vi "temperature-smoke-servo-control.vi"() -> ()   [LabVIEW 2019]
doc: "This example demonstrates how to read N channels of analog input from a LINX device."
uses:
  <vilib>/MakerHub/LINX/Public/Peripherals/Analog/Analog Read N Chans.vi
  <vilib>/MakerHub/LINX/Public/Peripherals/Analog/Analog Read 1 Chan.vi
  <vilib>/MakerHub/LINX/Public/Peripherals/Digital/Digital Write 1 Chan.vi
  <vilib>/MakerHub/LINX/Private/Local IO/LinxAnalogRead.vi
  <vilib>/MakerHub/LINX/Public/Utilities/Check Channel.vi
  <vilib>/MakerHub/LINX/Public/Peripherals/Digital/Digital Write N Chans.vi
  <vilib>/MakerHub/LINX/Private/Local IO/LinxDigitalWrite.vi
  <vilib>/MakerHub/LINX/Public/Utilities/Open Serial.vi
  <vilib>/MakerHub/LINX/Public/Sensors/Motion/Servo/Servo Open One Channel.vi
  <vilib>/MakerHub/LINX/Private/Utilties/Generate Error.vi
  <vilib>/imath/engines/lvmath2/RunTimeEngine/Managers/WorkSpace/UID Generator.vi
  <vilib>/imath/engines/lvmath2/RunTimeEngine/RunTimeType/NIMS_RunTimeType_From StrictType (excl LVString).vi
  <instcachedir>/0/NIMS_RunTimeType_From StrictType (excl LVString)_6DA94F09978249AAA8963F8D3C6FF051.lvgen/NIMS_RunTimeType_From StrictType (excl LVString)_6DA94F09978249AAA8963F8D3C6FF051_000.vi
  <vilib>/imath/engines/lvmath2/RunTimeEngine/LocalVariableDefStatement/MC_LocalVariableDefStatement_Display.vi
  <vilib>/imath/engines/lvmath2/RunTimeEngine/ArithmeticOperatorToken/NIMS_ArithmeticOperator_power(S).vi
  <instcachedir>/0/NIMS_ArithmeticOperator_power(S)_79C546042FF149A69349E20DC63C3C5B.lvgen/NIMS_ArithmeticOperator_power(S)_79C546042FF149A69349E20DC63C3C5B_014.vi
  <vilib>/imathl/engines/lvmath/Functions/Error Handling/Create Error.vi
  <vilib>/imath/engines/lvmath2/RunTimeEngine/Managers/SymbolTable/Clear UID.vi
  <vilib>/imath/engines/lvmath2/RunTimeEngine/NodeEndStatement/NIMS_NodeEndStatement_Output.vi
  <instcachedir>/0/NIMS_NodeEndStatement_Output_53EC0D466D134D7ABD903AC30B43404B.lvgen/NIMS_NodeEndStatement_Output_53EC0D466D134D7ABD903AC30B43404B_001.vi
  <instcachedir>/0/NIMS_NodeEndStatement_Output_53EC0D466D134D7ABD903AC30B43404B.lvgen/NIMS_NodeEndStatement_Output_53EC0D466D134D7ABD903AC30B43404B_008.vi
  <vilib>/imath/engines/lvmath2/RunTimeEngine/ErrorHandling/NIMS_Finalize Error.vi
  <instcachedir>/0/NIMS_NodeEndStatement_Output_53EC0D466D134D7ABD903AC30B43404B.lvgen/NIMS_NodeEndStatement_Output_53EC0D466D134D7ABD903AC30B43404B_010.vi
  <instcachedir>/0/NIMS_NodeEndStatement_Output_53EC0D466D134D7ABD903AC30B43404B.lvgen/NIMS_NodeEndStatement_Output_53EC0D466D134D7ABD903AC30B43404B_009.vi
  <vilib>/MakerHub/LINX/Public/Sensors/Motion/Servo/Servo Set Pulse Width One Channel.vi
  <vilib>/MakerHub/LINX/Public/Sensors/Motion/Servo/Servo Close One Channel.vi
  <vilib>/MakerHub/LINX/LMH-LINX.lvlib
  <vilib>/ptbypt/NI_PtbyPt.lvlib
  <vilib>/imath/engines/lvmath2/RunTimeEngine/Managers/SymbolTable/NIMS_WorkSpace.lvlib
  <vilib>/MakerHub/LINX/Public/Sensors/Motion/Servo/Servo.lvlib
panel:
  out "SERVO ANGLE":dbl(knob) scale=0.0..180.0
  out "V_SMOKE":dbl
  in  "Analog Channel (SMOKE)":u8
  in  "V_SMOKE MAX":dbl
  in  "Servo Channel":u8=2
  in  "V_SMOKE MIN":dbl
  out "DATA STORAGE STATUS":string
  in  "DATA STORAGE":bool
  out "WAVEFORM CHART":i32(graph)
  out "LOWER BAND":dbl
  out "UPPER BAND":dbl
  out "LIGHT LED":bool
  out "FAN LED":bool
  in  "SET TEMPERATURE RANGE":dbl
  in  "SET TEMPERATURE":dbl
  out "HUMIDITY":dbl(knob) scale=0.0..100.0
  out "TEMPERATURE":dbl(slide) scale=0.0..100.0
  in  "AI Channel(s)":u8[](array[numeric])=[0, 1, 2]
  in  "Stop Button":bool
  out "Loop Rate (Hz)":u32
  in  "Serial Port":refnum<visa-resource-name>
  # "LINX Device Settings"
  # "Analog Read N Channels Example (Serial Interface)\n\nThis example demonstrates how to read N channels of analog input values from a LINX device connected to the host computer via Serial / USB.\n\nInstructions\n1. Select the COM Port associated with the LINX Device.\n2. Select the Analog Channels to read.\n3. Click the Run Arrow."
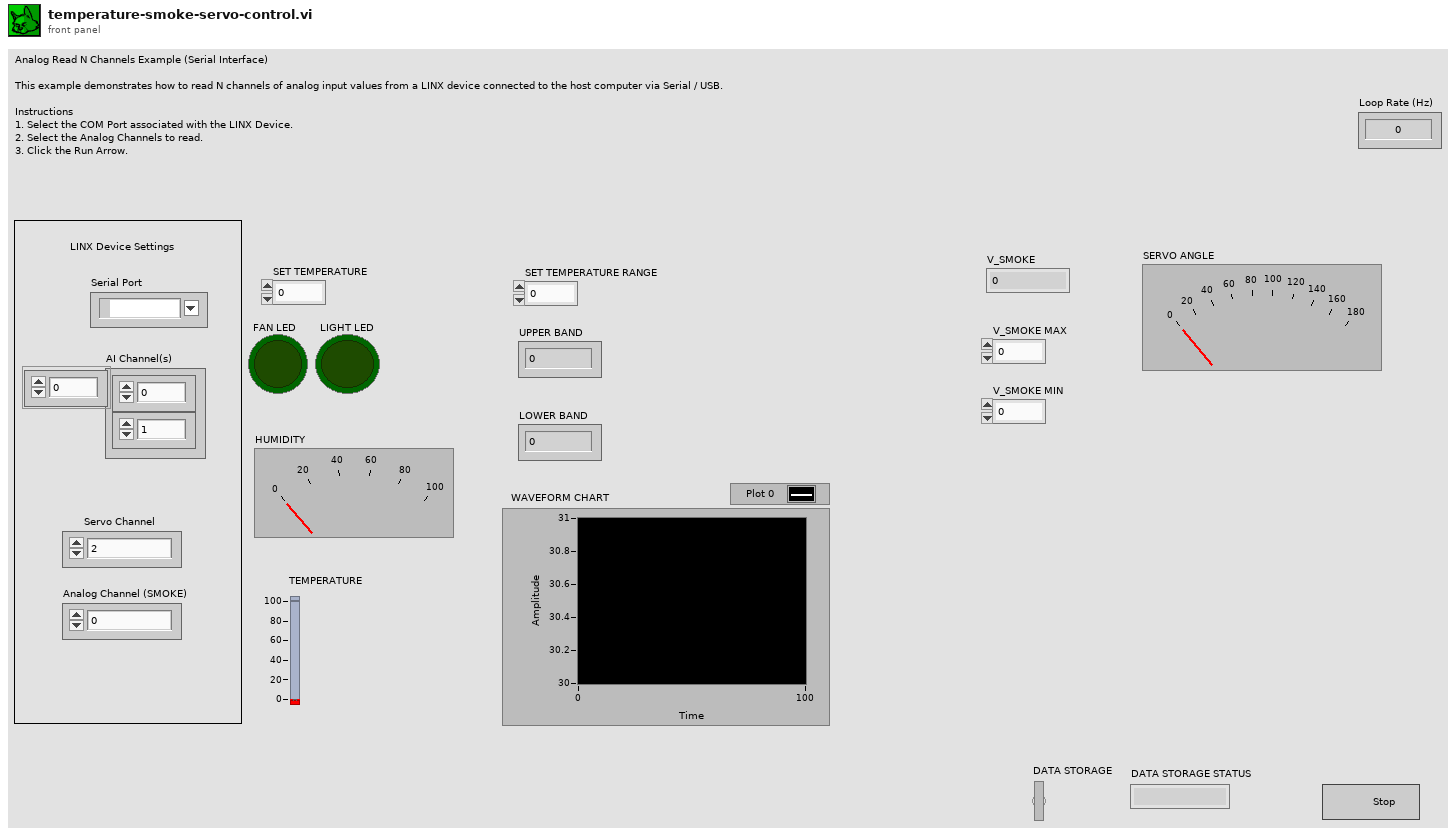
[diagram p1: front panel]
types:
  T1 = typedef "LMH-LINX.lvlib/LINX Ref.ctl" = cluster{"IO":T2, "Interface":T3, "LINX Device Config":T4}
  T2 = typedef "LMH-LINX.lvlib/Platform.ctl" = enum16{"Remote", "Local"}
  T3 = typedef "LMH-LINX.lvlib/Interface.ctl" = enum16{"Serial", "TCP"}
  T4 = typedef "LMH-LINX.lvlib/Device.lvlib/LINX Device Config.ctl" = cluster{"Interface":T3, "COM Port":refnum<visa-resource-name>, "TCP Configuration":T5, "Device Family":u8, "Device ID":u8, "Device Name":string, "TCP Ref":refnum<k5>, "Channels":T6}
  T5 = typedef "LMH-LINX.lvlib/Device.lvlib/TCP Config.ctl" = cluster{"IP Address":string, "Port":u16}
  T6 = typedef "LMH-LINX.lvlib/Channels.ctl" = cluster{"DI":u8[], "DO":u8[], "AI":u8[], "AO":u8[], "PWM":u8[], "QE":u8[], "UART":u8[], "I2C 2":u8[], "SPI":u8[], "CAN":u8[], "Servo":u8[], "AI Ref (V)":dbl, "AI Resolution (Bits)":u8, "AO Ref (V)":dbl, "AO Resolution (Bits)":u8}
  T7 = cluster{"Voltages[0]":dbl, "Voltages[1]":dbl, "Voltages[2]":dbl, "Voltages[3]":dbl, "Voltages[4]":dbl, "Voltages[5]":dbl, "Voltages[6]":dbl, "Voltages[7]":dbl, "Voltages[8]":dbl}
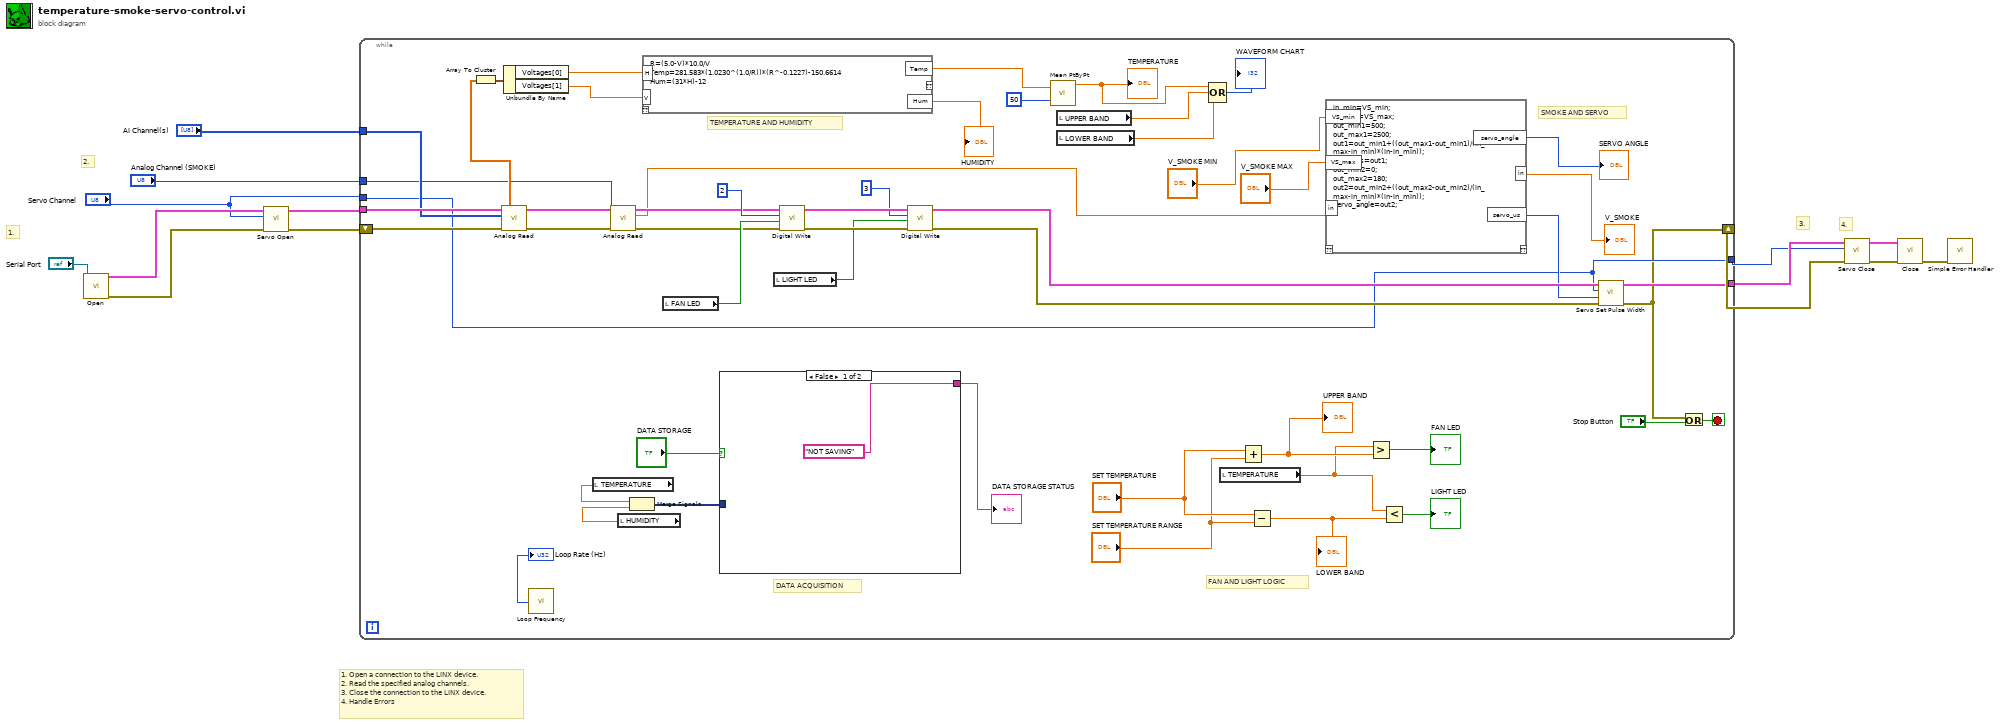
[diagram p0: block diagram]
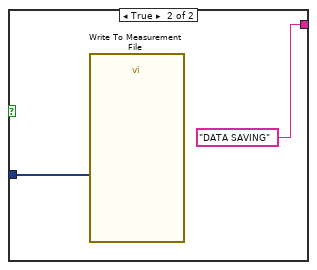
[diagram p2: hidden frame]
diagram:
  # "2."
  # "1. Open a connection to the LINX device.\n2. Read the specified analog channels.\n3. Close the connection to the LINX device.\n4. Handle Errors"
  # "4."
  # "3."
  # "1."
  n1 = call-poly <vilib>:"Open.vi"("Serial Port"="Serial Port") -> ("Error Out"=w9:errorcluster, "LINX Resource"=w11:T1)  [unwired: 8 in, 1 out]
  n2 = call-poly <vilib>:"Servo Open.vi"("Error In"=w9, "Servo Channel"="Servo Channel", "LINX Resource"=w11) -> ("Error Out"=w8:errorcluster, "LINX Resource"=w10:T1)  [unwired: 7 in]
  n3 = while {
    tunnel: w10 -> [w65]
    tunnel: [w21] -> w3
    shift-right: [w17] -> w5
    shift-left: w8 -> [w64]
    tunnel: "AI Channel(s)" -> [w41]
    tunnel: "Analog Channel (SMOKE)" -> [w26]
    tunnel: "Servo Channel" -> [w18]
    tunnel: [w18] -> w1
    stop <- w63 stop-if-true
    # "TEMPERATURE AND HUMIDITY"
    # "SMOKE AND SERVO"
    # "FAN AND LIGHT LOGIC"
    # "DATA ACQUISITION"
    n4 = call-poly <vilib>:"Analog Read.vi"("Error In"=w64, "AI Channel(s)"=w41, "LINX Resource"=w65) -> ("Error Out"=w29:errorcluster, "Voltages"=w60:dbl[], "LINX Resource"=w30:T1)  [unwired: 5 in, 1 out]
    n5 = Array To Cluster(array=w60) -> (cluster=w59:T7)
    n6 = Unbundle By Name(w59) -> ("Voltages[0]"=w58:dbl, "Voltages[1]"=w57:dbl)
    n7 = call <vilib>:"Loop Frequency.vi"() -> ("Loop Rate (Hz)"=→"Loop Rate (Hz)":u32)
    n8 = local read "TEMPERATURE"() -> (w37:dbl)
    n9 = call-poly <vilib>:"Analog Read.vi"("Error In"=w29, "Analog Channel"=w26, "LINX Resource"=w30) -> ("Error Out"=w28:errorcluster, "Voltage"=w25:dbl, "LINX Resource"=w27:T1)  [unwired: 5 in, 1 out]
    n10 = local read "HUMIDITY"() -> (w36:dbl)
    n11 = Merge Signals(w37, w36) -> (w35:dynamicdata)
    n12 = mathscript code="R=(5.0-V)*10.0/V\nTemp=281.583*(1.0230^(1.0/R))*(R^-0.1227)-150.6614\nHum=(31*H)-12"("H"=w58, "V"=w57) -> ("Temp"=w44:cdb, "Hum"=→"HUMIDITY":dbl)  [unwired: 1 in, 1 out]
    n13 = local read "FAN LED"() -> (w46:bool)
    n14 = case shown="False" "DATA STORAGE" {
      tunnel: w35 -> [_ w157]
      tunnel: ["NOT SAVING" "DATA SAVING"] -> w33
      frame False {
      }
      frame True {
        n15 = call "Write To Measurement File"("Signals"=w157) -> ()  [unwired: 16 in, 3 out]
      }
    }
    "DATA STORAGE STATUS" <- w33
    n16 = local read "LIGHT LED"() -> (w45:bool)
    n17 = call-poly <vilib>:"Digital Write.vi"("Error In"=w28, "Output Value"=w46, "DO Channel"=u8 2, "LINX Resource"=w27) -> ("Error Out"=w54:errorcluster, "LINX Resource"=w55:T1)  [unwired: 6 in]
    n18 = call-poly <vilib>:"Digital Write.vi"("Error In"=w54, "Output Value"=w45, "DO Channel"=u8 3, "LINX Resource"=w55) -> ("Error Out"=w20:errorcluster, "LINX Resource"=w22:T1)  [unwired: 6 in]
    n19 = call <vilib>:"Mean PtByPt.vi"("x"=w44, "sample length"=50) -> ("mean"=w40:dbl)  [unwired: 2 in, 1 out]
    "TEMPERATURE" <- w40
    n20 = local read "UPPER BAND"() -> (w39:dbl)
    n21 = local read "LOWER BAND"() -> (w38:dbl)
    n22 = Compound Arithmetic op=OR(w40, w39, w38) -> (→"WAVEFORM CHART":i32)
    n23 = local read "TEMPERATURE"() -> (w50:dbl)
    n24 = Add(x="SET TEMPERATURE", y="SET TEMPERATURE RANGE") -> (x+y=w51:dbl)
    "UPPER BAND" <- w51
    n25 = Subtract(x="SET TEMPERATURE", y="SET TEMPERATURE RANGE") -> (x-y=w49:dbl)
    "LOWER BAND" <- w49
    n26 = mathscript code="in_min=VS_min;\nin_max=VS_max;\nout_min1=500;\nout_max1=2500;\nout1=out_min1+((out_max1-out_min1)/(in_max-in_min)*(in-in_min));\nservo_us=out1;\nout_min2=0;\nout_max2=180;\nout2=out_min2+((out_max2-out_min2)/(in_max-in_min)*(in-in_min));\nservo_angle=out2;"("in"=w25, "VS_min"="V_SMOKE MIN", "VS_max"="V_SMOKE MAX") -> ("servo_us"=w19:i32, "servo_angle"=→"SERVO ANGLE":i64, "in"=→"V_SMOKE":dbl)  [unwired: 1 in, 1 out]
    n27 = Greater?(x=w50, y=w51) -> (0:→"FAN LED":bool)
    n28 = Less?(x=w50, y=w49) -> (x < y?=→"LIGHT LED":bool)
    n29 = call-poly <vilib>:"Servo Set Pulse Width.vi"("Error In"=w20, "Pulse Width (uS)"=w19, "Servo Channel"=w18, "LINX Resource"=w22) -> ("Error Out"=w17:errorcluster, "LINX Resource"=w21:T1)  [unwired: 6 in]
    n30 = Or(x=w17, y="Stop Button") -> (x .or. y?=w63:bool)
  }
  n31 = call-poly <vilib>:"Servo Close.vi"("Error In"=w5, "Servo Channel"=w1, "LINX Resource"=w3) -> ("Error Out"=w4:errorcluster, "LINX Resource"=w2:T1)  [unwired: 7 in]
  n32 = call <vilib>:"Close.vi"("Error In"=w4, "LINX Resource"=w2) -> ("Error Out"=w13:errorcluster)  [unwired: 9 in]
  n33 = call <vilib>:"Simple Error Handler.vi"("error in (no error)"=w13) -> ()  [unwired: 4 in, 5 out]
